vi "Periodic Tasks.vi"(8 "error in":errorcluster) -> ()   [LabVIEW 2011]
doc: "This VI runs in parallel to other tasks. It can contain as many user-defined periodic loops as you need. These can carry out PID or other sorts of timed response."
uses:
  <vilib>/Rock Robotics/SystemInterfaces/Utilities/FPGA_UtilitiesLED State.ctl
  <vilib>/Rock Robotics/SystemInterfaces/Utilities/FPGA_UtilitiesLED Source.ctl
  Robot Global Data.vi
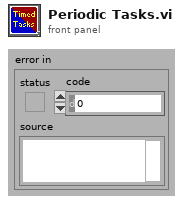
[diagram p1: front panel]
types:
  T1 = typedef "FPGA_UtilitiesLED State.ctl" = enum16{"Off", "On", "Toggle"}
  T2 = typedef "FPGA_UtilitiesLED Source.ctl" = enum16{"User LED", "FPGA LED"}
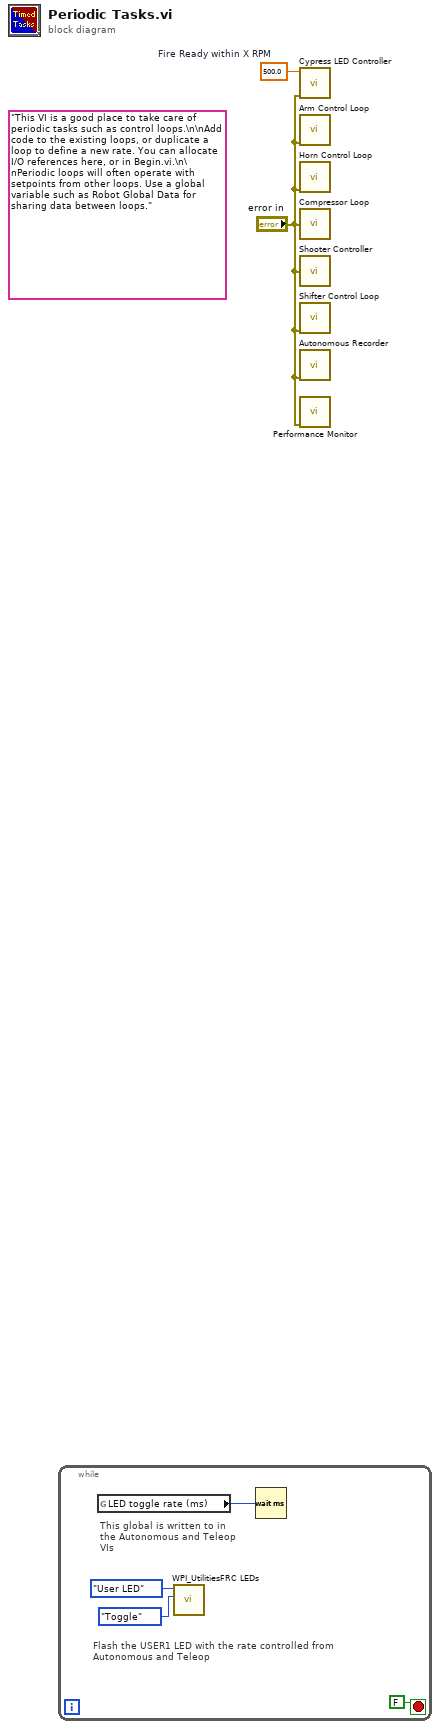
[diagram p0: block diagram]
diagram:
  w2 = 500.0  # Fire Ready within X RPM
  (unwired) "This VI is a good place to take care of periodic tasks such as control loops.\n\nAdd code to the existing loops, or duplicate a loop to define a new rate. You can allocate I/O references here, or in Begin.vi.\n\nPeriodic loops will often operate with setpoints from other loops. Use a global variable such as Robot Global Data for sharing data between loops."
  n1 = while {
    stop <- FALSE stop-if-true
    # "This global is written to in the Autonomous and Teleop VIs"
    # "Flash the USER1 LED with the rate controlled from Autonomous and Teleop"
    n2 = global read "Robot Global Data.vi" "LED toggle rate (ms)"() -> (w3:u32)
    n3 = call <vilib>:"WPI_UtilitiesFRC LEDs.vi"("State"=FPGA_UtilitiesLED_State."Toggle", "LED Type"=FPGA_UtilitiesLED_Source."User LED") -> ()  [unwired: 1 in, 9 out]
    n4 = Wait (ms)(milliseconds to wait=w3) -> ()  [unwired: 1 out]
  }
  n5 = call "Cypress LED Controller.vi"("error in (no error)"="error in", "Fire Ready within X RPM"=w2) -> ()  [unwired: 10 in]
  n6 = call "Arm Control Loop.vi"("error in (no error)"="error in") -> ()  [unwired: 11 in]
  n7 = call "Horn Control Loop.vi"("error in (no error)"="error in") -> ()  [unwired: 11 in]
  n8 = call "Compressor Loop.vi"("error in (no error)"="error in") -> ()
  n9 = call "Shooter Controller.vi"("error in (no error)"="error in") -> ()
  n10 = call "Shifter Control Loop.vi"("error in (no error)"="error in") -> ()  [unwired: 11 in]
  n11 = call "Autonomous Recorder.vi"("error in (no error)"="error in") -> ()  [unwired: 11 in]
  n12 = call "Performance Monitor.vi"("error in (no error)"="error in") -> ()  [unwired: 11 in]
